vi "QTrkCUDA_EnableTextureCache.vi"() -> ()   [LabVIEW 2011]
uses:
  QTrkInstance.ctl
  QTrkDLL.vi
panel:
  in  "Enable? (T)":bool=TRUE
  out "error out":errorcluster
  in  "error in (no error)":errorcluster
  in  "QTrk Instance":T1
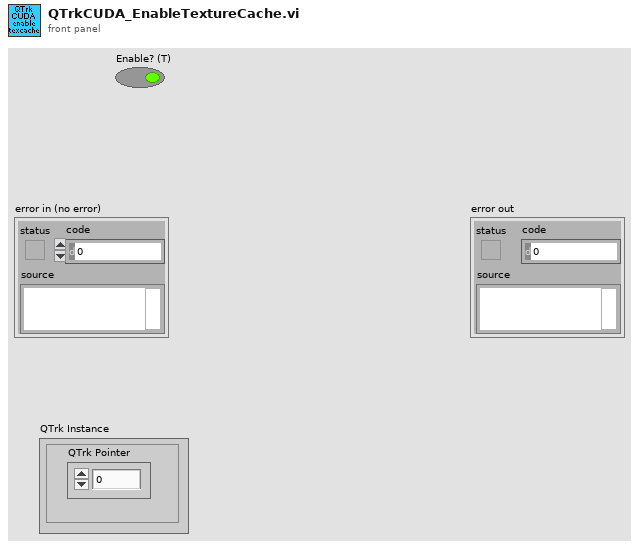
[diagram p1: front panel]
types:
  T1 = typedef "QTrkInstance.ctl" = cluster{"QTrk Pointer":u64}
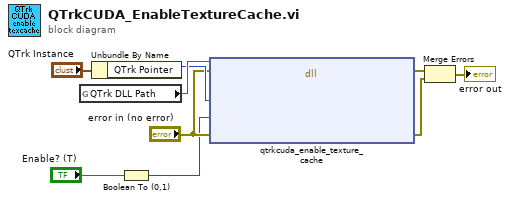
[diagram p0: block diagram]
diagram:
  n1 = global read "QTrkDLL.vi" "QTrk DLL Path"() -> (w9:path)
  n2 = Unbundle By Name("QTrk Instance") -> ("QTrk Pointer"=w7:u64)
  n3 = Boolean To (0,1)(Boolean="Enable? (T)") -> (0, 1=w1:i16)
  n4 = dll-call lib="D:/jcnossen1/cudaqi-tracker/cudatrack-labview/cputrack_d.dll" fn="qtrkcuda_enable_texture_cache"(path in=w9, error in="error in (no error)", "instance"=w7, "enable"=w1, "error"="error in (no error)") -> (error out=w5:errorcluster, "error"=w4:errorcluster)  [unwired: 4 in, 1 out]
  n5 = Merge Errors(w5, w4) -> (→"error out":errorcluster)
